vi "Server_Load Data Log.vi"(8 "error in":errorcluster, 11 "User Name":string) -> (0 "error out":errorcluster, 3 "Log Data":T1[](array[typedef]))   [LabVIEW 2018, in "Cloud Server.lvlib"]
uses:
  Cloud Server.lvlib
  Com VIs/Data Def/Data File Format.ctl
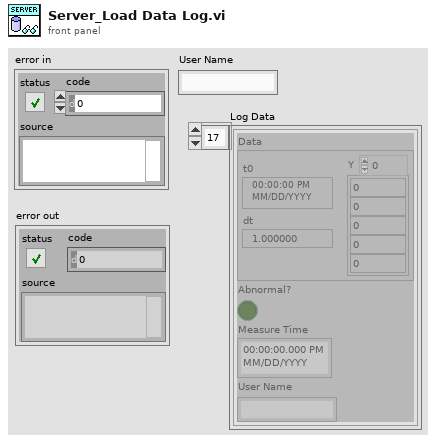
[diagram p1: front panel]
types:
  T1 = typedef "Data File Format.ctl" = cluster{"Data":waveform(dbl), "Abnormal?":bool, "Measure Time":timestamp, "User Name":string}
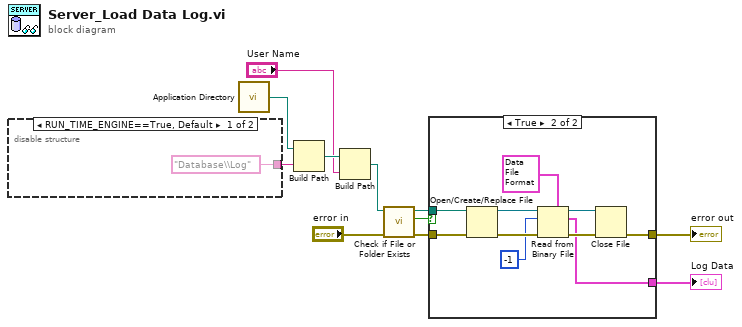
[diagram p0: block diagram]
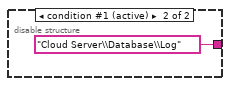
[diagram p3: hidden frame]
diagram:
  n1 = disable-structure shown="RUN_TIME_ENGINE==True, Default" {
    disable-tunnel: ["Database\\Log" ("name or relative path") "Cloud Server\\Database\\Log" ("name or relative path")] -> w11
    frame condition #0 {
    }
    frame condition #1 (active) {
    }
  }
  n2 = call <vilib>:"Application Directory.vi"() -> ("Application Directory"=w10:path)
  n3 = Build Path(base path=w10, name or relative path=w11) -> (appended path=w9:path)
  n4 = Build Path(base path=w9, name or relative path="User Name") -> (appended path=w3:path)
  n5 = call <vilib>:"Check if File or Folder Exists.vi"("error in (no error)"="error in", "path"=w3) -> ("error out"=w5:errorcluster, "file or folder exists?"=w2:bool, "dup path"=w1:path)  [unwired: 7 in]
  n6 = case shown="True" w2 {
    tunnel: [w14 w18] -> w7
    tunnel: [_ w17] -> w6
    tunnel: w5 -> [w14 w16]
    tunnel: w1 -> [_ w15]
    frame False {
    }
    frame True {
      n7 = Open/Create/Replace File(file path (use dialog)=w15, error in=w16) -> (refnum out=w23:refnum<file>, error out=w24:errorcluster)  [unwired: 4 in, 1 out]
      n8 = Read from Binary File(5:T1 {"Data"={"t0"=timestamp(0 s since 1904-01-01), "dt"=1.0, "Y"=[]}, "Abnormal?"=FALSE, "Measure Time"=timestamp(0 s since 1904-01-01), "User Name"=""} ("Data File Format"), 8:w24, 10:-1 ("count (1)"), 11:w23) -> (0:w20:errorcluster, 2:w17:T1[], 3:w19:refnum<file>)  [unwired: 2 in, 1 out]
      n9 = Close File(refnum=w19, error in=w20) -> (error out=w18:errorcluster)  [unwired: 1 out]
    }
  }
  "error out" <- w7
  "Log Data" <- w6
